vi "字符串转utf-8.vi"(8 "错误输入":errorcluster, 11 "文本":string) -> (0 "错误输出":errorcluster, 3 "utf-8文本":string)   [LabVIEW 2017]
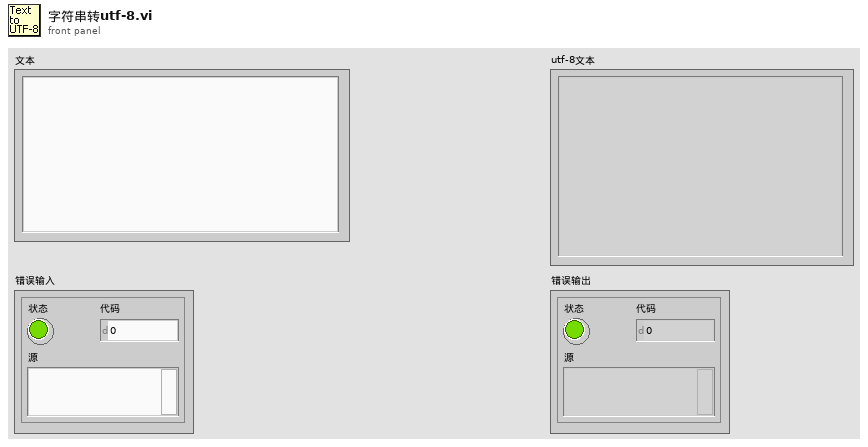
[diagram p1: front panel]
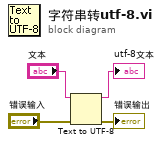
[diagram p0: block diagram]
diagram:
  n1 = Text to UTF-8(8:"错误输入", 11:"文本") -> (0:→"错误输出":errorcluster, 3:→"utf-8文本":string)  [unwired: 1 in]
